vi "Sea-Level SWI Unflatten Driver Configuration.vi"(9 "SWI Configuration (\"\")":string) -> (1 "Configuration":T1, 4 "Version":string)   [LabVIEW 2011]
uses:
  TypeDefs/Sea-Level SWI Configuration.ctl
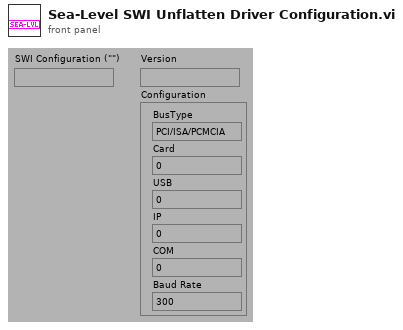
[diagram p1: front panel]
types:
  T1 = typedef "Sea-Level SWI Configuration.ctl" = cluster{"BusType":enum32{"PCI/ISA/PCMCIA", "USB", "Ethernet", "Serial"}, "Card":i32, "USB":i32, "IP":u32, "COM":i32, "Baud Rate":enum16{"300", "600", "1200", "2400", "4800", "9600"}}
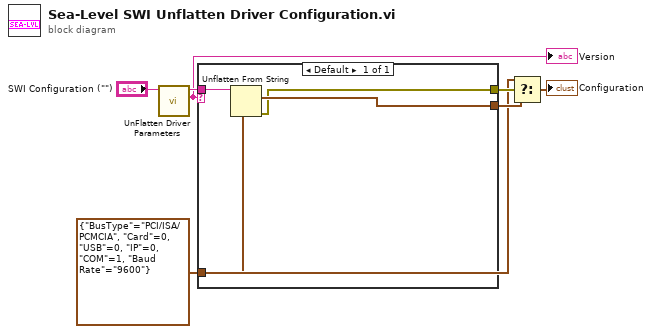
[diagram p0: block diagram]
diagram:
  w1 = T1 {"BusType"=enum."PCI/ISA/PCMCIA", "Card"=0, "USB"=0, "IP"=0, "COM"=1, "Baud Rate"=enum."9600"} ("Configuration")
  n1 = call "UnFlatten Driver Parameters.vi"("Flattened Driver Parameters with Version (\"\")"="SWI Configuration (\"\")") -> ("Driver Version"=w2:string, "Flat Driver Parameters"=w3:string)  [unwired: 1 in, 4 out]
  "Version" <- w2
  n2 = case shown="Default" w2 {
    tunnel: [w11] -> w7
    tunnel: [w8] -> w5
    tunnel: w3 -> [w10]
    tunnel: w1 -> [w9]
    frame Default {
      n3 = Unflatten From String(type=w9, binary string=w10) -> (value=w11:T1, error out=w8:errorcluster)  [unwired: 1 in, 3 out]
    }
  }
  n4 = Select(t=w1, s=w5, f=w7) -> (s? t:f=→"Configuration":T1)
